vi "Send Ping.vi"(6 "Return Self (F)":bool, 7 "Message Priority (Normal)":T1=enum."Normal", 8 "error in (no error)":errorcluster, 9 "timeout in ms (1000)":i32=1000, 11 "Message Enqueuer":refnum<class "Message Enqueuer.lvclass">) -> (0 "error out":errorcluster, 1 "timed out?":bool, 2 "Actor out":refnum<class "Actor.lvclass">, 3 "Message Enqueuer out":refnum<class "Message Enqueuer.lvclass">)   [LabVIEW 2015, in "cRIO-Carbondioxide.lvlib" / "CO2-Actor.lvlib" / "Ping Msg.lvclass"]
doc: "This VI sends the message to an actor."
uses:
  Ping Msg.lvclass
  <vilib>/ActorFramework/Message Enqueuer/Message Enqueuer.lvclass
  <vilib>/ActorFramework/Message Enqueuer/Message Priority.ctl
  <vilib>/ActorFramework/Actor/Actor.lvclass
  Ping Msg.lvclass/Ping Msg.ctl
  <vilib>/ActorFramework/Message Enqueuer/Message Enqueuer.lvclass/Message Enqueuer.ctl
  <vilib>/ActorFramework/Message Priority Queue/Priority Enqueue.vi
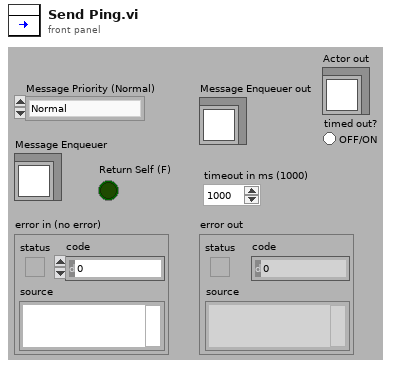
[diagram p1: front panel]
types:
  T1 = typedef "Actor Framework.lvlib/Message Enqueuer.lvclass/Message Priority.ctl" = enum16{"Low", "Normal", "High"}
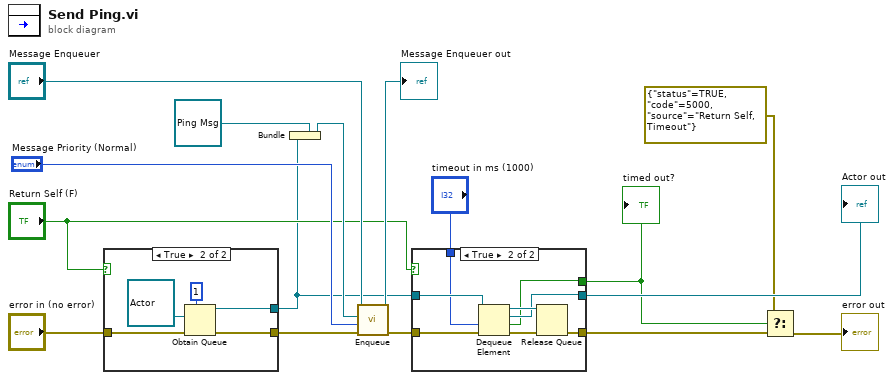
[diagram p0: block diagram]
diagram:
  n1 = case shown="True" "Return Self (F)" {
    tunnel: "error in (no error)" -> [w17 w20]
    tunnel: [w17 w19] -> w12
    tunnel: [_ w18] -> w7
    frame False {
    }
    frame True {
      n2 = Obtain Queue(max queue size (-1, unlimited)=1, element data type=refnum<class "Actor.lvclass"> refnum ("Actor"), error in (no error)=w20) -> (queue out=w18:refnum<queue>, error out=w19:errorcluster)  [unwired: 2 in, 1 out]
    }
  }
  n3 = Bundle(cluster=refnum<class "Ping Msg.lvclass"> refnum ("Object"), w7) -> (w11:refnum<class "Ping Msg.lvclass">)
  n4 = call <vilib>:"Enqueue.vi"("error in (no error)"=w12, "Message Priority (Normal)"="Message Priority (Normal)", "Message"=w11, "Message Enqueuer in"="Message Enqueuer") -> ("error out"=w9:errorcluster, "Message Enqueuer out"=→"Message Enqueuer out":refnum<class "Message Enqueuer.lvclass">)  [unwired: 6 in]
  n5 = case shown="True" "Return Self (F)" {
    tunnel: w9 -> [w23 w31]
    tunnel: [w23 w27] -> w4
    tunnel: w7 -> [_ w30]
    tunnel: "timeout in ms (1000)" -> [_ w29]
    tunnel: [_ w25] -> w5
    tunnel: [_ w24] -> w2
    frame False {
    }
    frame True {
      n6 = Dequeue Element(queue=w30, timeout in ms (-1)=w29, error in (no error)=w31) -> (queue out=w26:refnum<queue>, element=w25:refnum<class "Actor.lvclass">, timed out?=w24:bool, error out=w28:errorcluster)
      n7 = Release Queue(queue=w26, error in (no error)=w28) -> (error out=w27:errorcluster)  [unwired: 1 in, 2 out]
    }
  }
  "Actor out" <- w5
  "timed out?" <- w2
  n8 = Select(t=errorcluster {"status"=TRUE, "code"=5000, "source"="Return Self, Timeout"} ("error constant"), s=w2, f=w4) -> (s? t:f=→"error out":errorcluster)
